vi "Specify Feed Settings Dialog.vi"(11 "error in (no error)":errorcluster) -> (4 "feed name out":string, 6 "feed folderpath out":path, 8 "package destination folderpath out":path, 10 "cancelled?":bool, 15 "error out":errorcluster)   [LabVIEW 2014]
doc: "This VI launches a dialog that prompts the user to add a feed to manage."
uses:
  <vilib>/National Instruments/NIPM API (Beta)/NIPM_API.lvlib
  Specify Feed Settings States.ctl
panel:
  in  "Package Destination Folderpath":path
  in  "Use feed folderpath":bool=TRUE
  in  "Cancel":bool
  in  "OK":bool
  in  "Feed Folderpath":path
  in  "Feed Name":string
  # "Package Destination Folderpath"
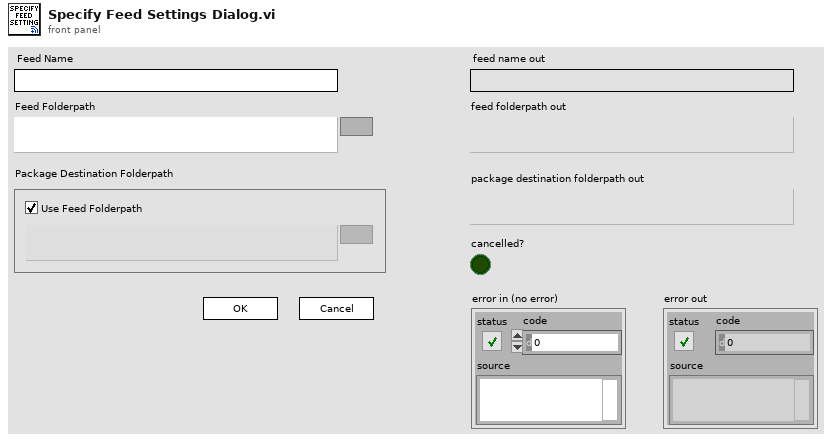
[diagram p1: front panel]
types:
  T1 = typedef "Specify Feed Settings States.ctl" = enum16{"Initialize", "Wait for Event", "Update Display", "Exit"}
  T2 = enum8{"Enabled", "Disabled", "Disabled and Grayed Out"}
  T3 = cluster{"Feed Name":string, "Feed Folderpath":path, "Package Destination Folderpath":path, "Use feed folderpath":bool, "cancelled?":bool}
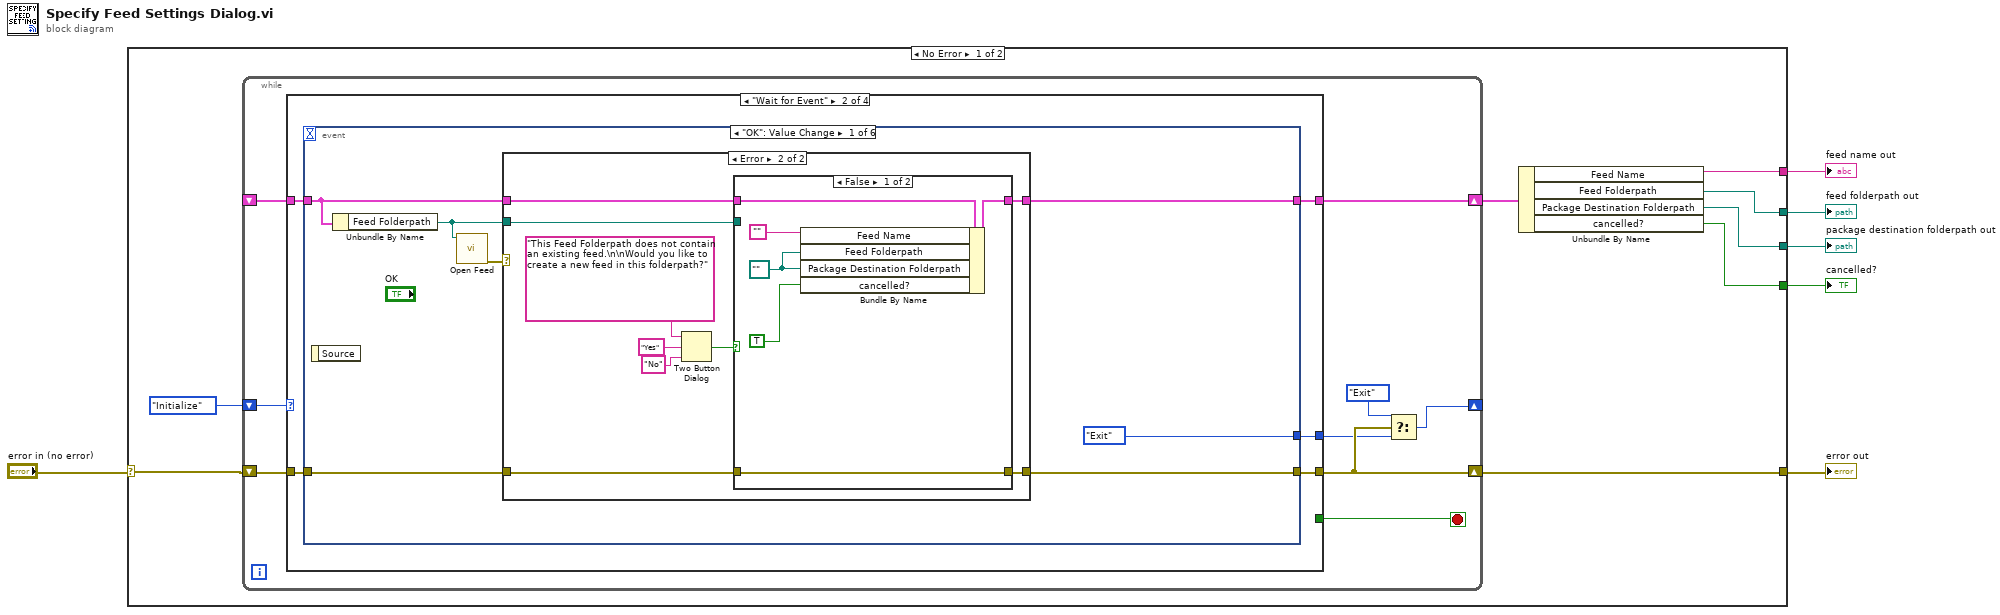
[diagram p0: block diagram]
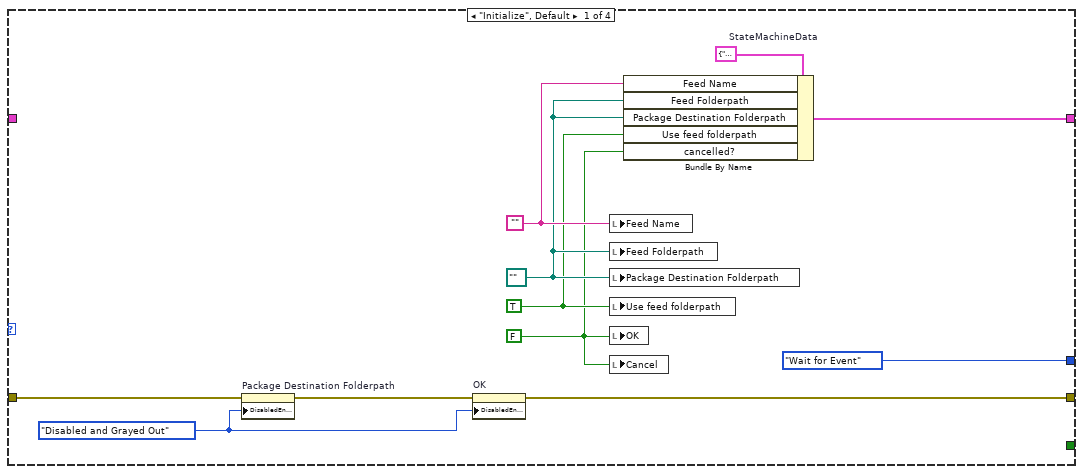
[diagram p2: hidden frame]
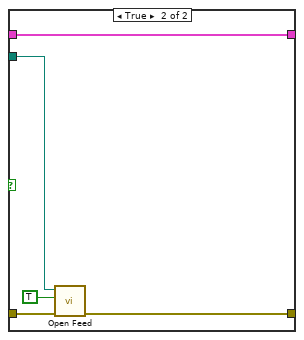
[diagram p4: hidden frame]
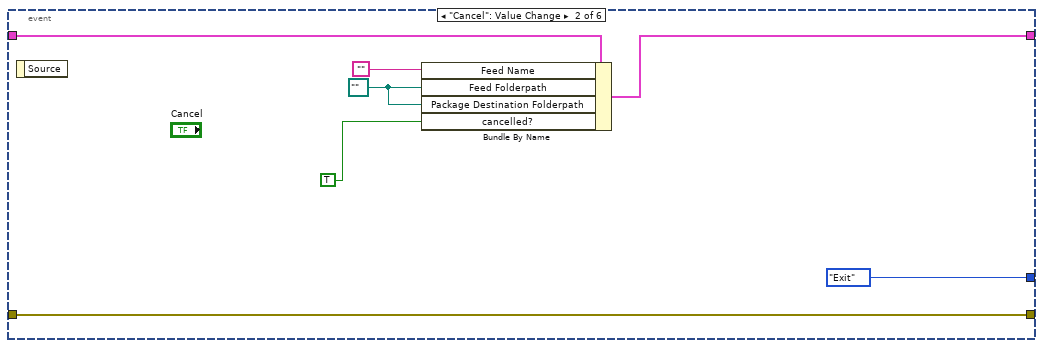
[diagram p5: hidden frame]
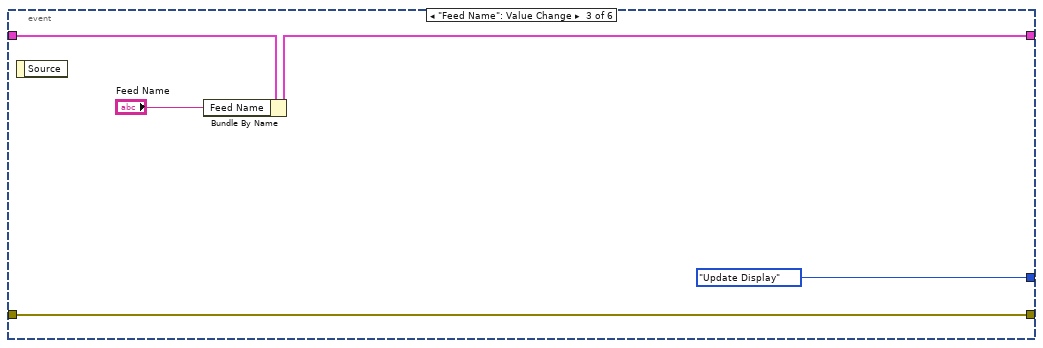
[diagram p6: hidden frame]
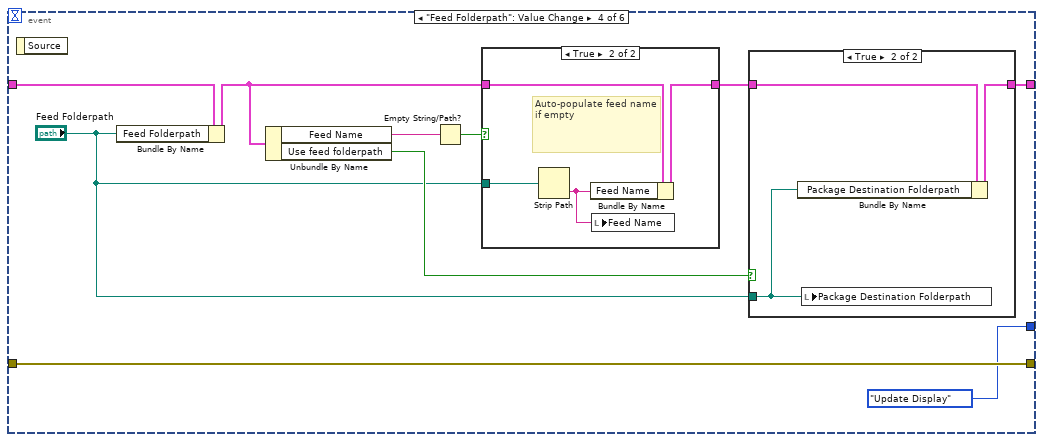
[diagram p7: hidden frame]
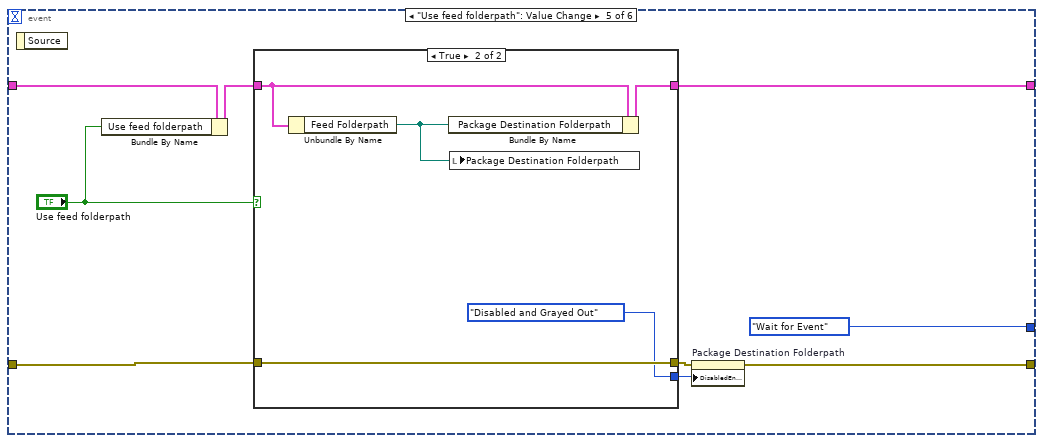
[diagram p10: hidden frame]
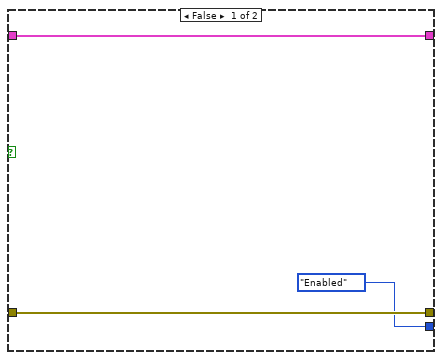
[diagram p11: hidden frame]
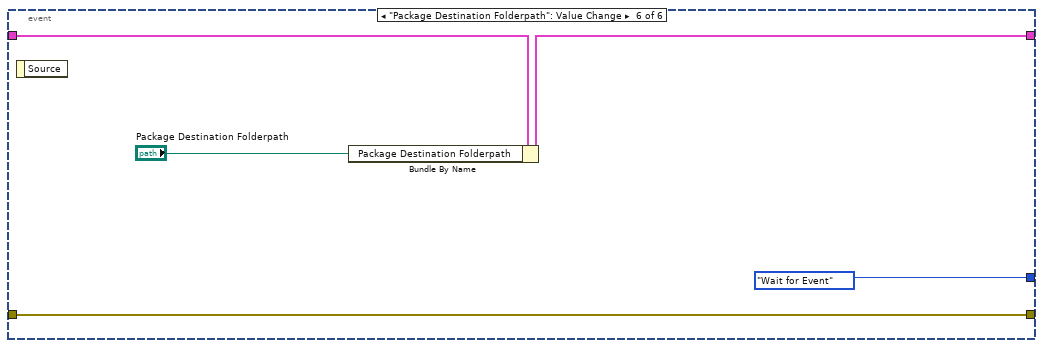
[diagram p12: hidden frame]
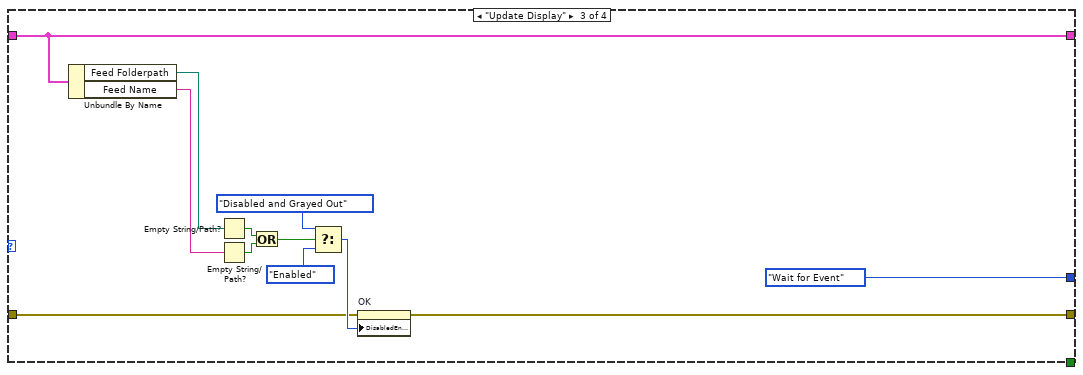
[diagram p13: hidden frame]
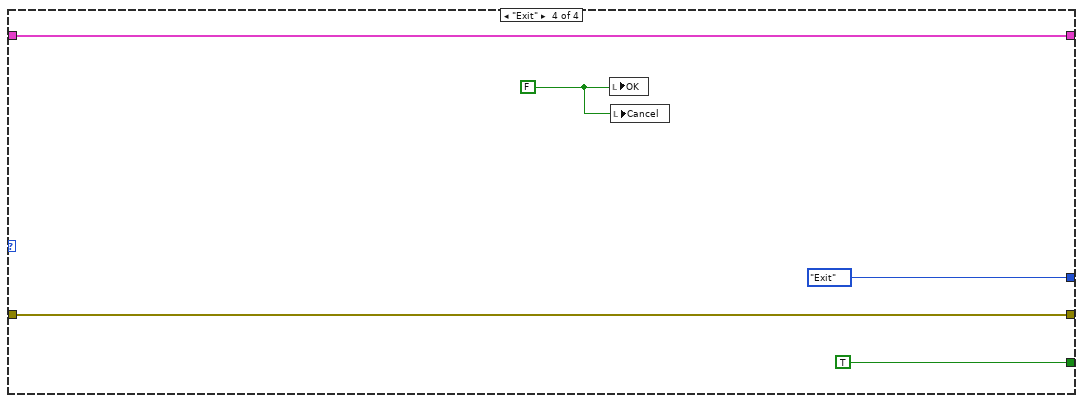
[diagram p14: hidden frame]
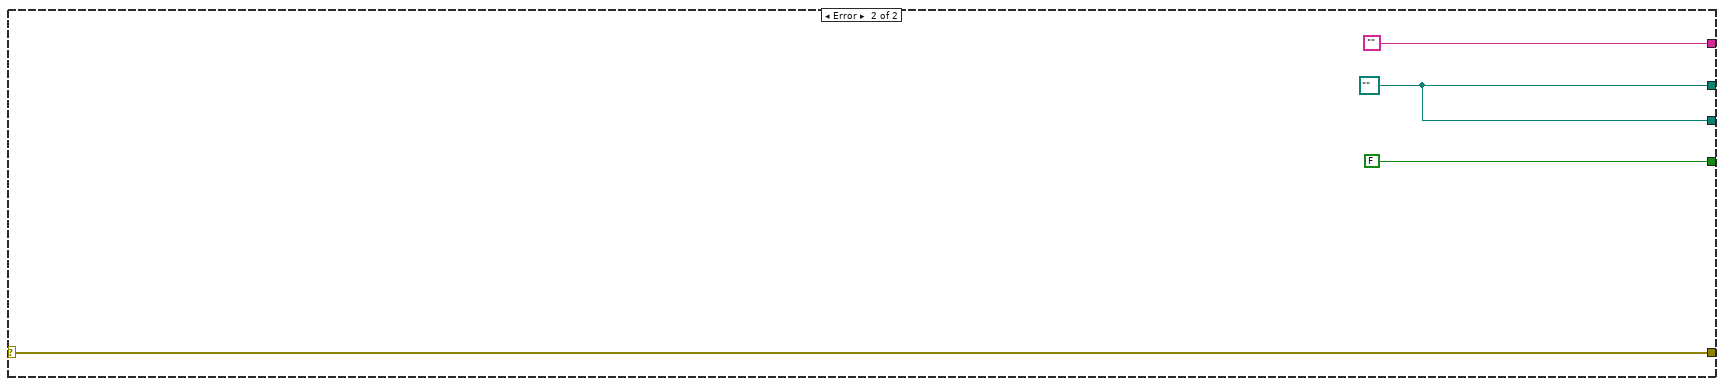
[diagram p15: hidden frame]
diagram:
  n1 = case shown="No Error" "error in (no error)" {
    selector: "error in (no error)" -> [w8 w142]
    tunnel: [w10 FALSE] -> w6
    tunnel: [w12 w139] -> w5
    tunnel: [w11 w139] -> w1
    tunnel: [w14 w142] -> w3
    tunnel: [w7 "" ("Feed Name")] -> w2
    frame No Error {
      n2 = while {
        shift-right: [w18] -> w14
        shift-left: w8 -> [w21]
        shift-right: [w22] -> w13
        shift-left: _ -> [w23]
        shift-right: [w16] -> _
        shift-left: Specify_Feed_Settings_States."Initialize" -> [w20]
        stop <- w19 stop-if-true
        n3 = case shown="\"Wait for Event\"" w20 {
          tunnel: [_ _ _ TRUE] -> w19
          tunnel: w23 -> [_ w39 w125 w136]
          tunnel: [w24 w38 w125 w136] -> w22
          tunnel: w21 -> [w33 w37 w124 w135]
          tunnel: [w30 w36 w123 w135] -> w18
          tunnel: [Specify_Feed_Settings_States."Wait for Event" w35 Specify_Feed_Settings_States."Wait for Event" Specify_Feed_Settings_States."Exit"] -> w15
          frame "Initialize", Default {
            w25 = FALSE ("Use feed folderpath")
            w29 = T3 {"Feed Name"="", "Feed Folderpath"=path "", "Package Destination Folderpath"=path "", "Use feed folderpath"=FALSE, "cancelled?"=FALSE}  # StateMachineData
            w28 = "" ("Feed Name")
            w27 = path "" ("Package Destination Folderpath")
            w26 = TRUE ("Use feed folderpath")
            w31 = T2."Disabled and Grayed Out" ("Disabled")
            n4 = property on="Package Destination Folderpath" class="Path"(error in=w33, "DisabledEnum"=w31) -> (error out=w32:errorcluster)  [unwired: 1 in, 1 out]
            n5 = property on="OK" class="Bool (strict)"(error in=w32, "DisabledEnum"=w31) -> (error out=w30:errorcluster)  [unwired: 1 in, 1 out]
            n6 = local write "Feed Name"(w28) -> ()
            n7 = local write "Feed Folderpath"(w27) -> ()
            n8 = local write "Package Destination Folderpath"(w27) -> ()
            n9 = local write "Use feed folderpath"(w26) -> ()
            n10 = local write "OK"(w25) -> ()
            n11 = local write "Cancel"(w25) -> ()
            n12 = Bundle By Name(cluster=w29, "Feed Name"=w28, "Feed Folderpath"=w27, "Package Destination Folderpath"=w27, "Use feed folderpath"=w26, "cancelled?"=w25) -> (w24:T3)
          }
          frame "Wait for Event" {
            n13 = event shown="[0] \"OK\": Value Change" {
              selector: _ -> [_ _ _ _ _ _]
              dyn-events: _ -> [_ _ _ _ _ _]
              timeout: _ -> [_ _ _ _ _ _]
              tunnel: w39 -> [w45 w75 w80 w90 w108 w121]
              tunnel: [w44 w74 w79 w81 w105 w119] -> w38
              tunnel: w37 -> [w42 w72 w77 w86 w104 w120]
              tunnel: [w41 w72 w77 w86 w107 w120] -> w36
              tunnel: [Specify_Feed_Settings_States."Exit" Specify_Feed_Settings_States."Exit" Specify_Feed_Settings_States."Update Display" Specify_Feed_Settings_States."Update Display" Specify_Feed_Settings_States."Wait for Event" Specify_Feed_Settings_States."Wait for Event"] -> w35
              event "OK": Value Change {
                n14 = event-data() -> ()  [unwired: 1 in, 1 out]
                n15 = Unbundle By Name(w45) -> ("Feed Folderpath"=w43:path)
                n16 = call <vilib>:"Open Feed.vi"("feed folderpath"=w43) -> ("error out"=w46:errorcluster)  [unwired: 8 in, 2 out]
                n17 = case shown="Error" w46 {
                  tunnel: w45 -> [w48 w53]
                  tunnel: [w48 w52] -> w44
                  tunnel: w43 -> [_ w51]
                  tunnel: w42 -> [w47 w50]
                  tunnel: [w47 w49] -> w41
                  frame No Error {
                  }
                  frame Error {
                    n18 = Two Button Dialog(message="This Feed Folderpath does not contain an existing feed.\n\nWould you like to create a new feed in this folderpath?", 1:"No" ("F button name (\"Cancel\")"), 2:"Yes" ("T button name (\"OK\")")) -> (T button?=w54:bool)
                    n19 = case shown="False" w54 {
                      tunnel: w53 -> [w62 w67]
                      tunnel: [w61 w67] -> w52
                      tunnel: w51 -> [_ w66]
                      tunnel: w50 -> [w63 w65]
                      tunnel: [w63 w64] -> w49
                      frame False {
                        w59 = path "" ("Feed Folderpath")
                        n20 = Bundle By Name(cluster=w62, "Feed Name"="", "Feed Folderpath"=w59, "Package Destination Folderpath"=w59, "cancelled?"=TRUE) -> (w61:T3)
                      }
                      frame True {
                        n21 = call <vilib>:"Open Feed.vi"("error in"=w65, "create feed if necessary (F)"=TRUE, "feed folderpath"=w66) -> ("error out"=w64:errorcluster)  [unwired: 6 in, 2 out]
                      }
                    }
                  }
                }
              }
              event "Cancel": Value Change {
                w70 = path "" ("Feed Folderpath")
                n22 = event-data() -> ()  [unwired: 1 in, 1 out]
                n23 = Bundle By Name(cluster=w75, "Feed Name"="", "Feed Folderpath"=w70, "Package Destination Folderpath"=w70, "cancelled?"=TRUE) -> (w74:T3)
              }
              event "Feed Name": Value Change {
                n24 = event-data() -> ()  [unwired: 1 in, 1 out]
                n25 = Bundle By Name(cluster=w80, "Feed Name"="Feed Name") -> (w79:T3)
              }
              event "Feed Folderpath": Value Change {
                n26 = event-data() -> ()  [unwired: 1 in, 1 out]
                n27 = Bundle By Name(cluster=w90, "Feed Folderpath"="Feed Folderpath") -> (w88:T3)
                n28 = Unbundle By Name(w88) -> ("Feed Name"=w89:string, "Use feed folderpath"=w84:bool)
                n29 = Empty String/Path?(string/path=w89) -> (empty?=w87:bool)
                n30 = case shown="True" w87 {
                  tunnel: [w95 w98] -> w82
                  tunnel: w88 -> [w95 w99]
                  tunnel: "Feed Folderpath" -> [_ w97]
                  frame False {
                  }
                  frame True {
                    # "Auto-populate feed name if empty"
                    n31 = Strip Path(path=w97) -> (name=w96:string)  [unwired: 1 out]
                    n32 = Bundle By Name(cluster=w99, "Feed Name"=w96) -> (w98:T3)
                    n33 = local write "Feed Name"(w96) -> ()
                  }
                }
                n34 = case shown="True" w84 {
                  tunnel: "Feed Folderpath" -> [_ w92]
                  tunnel: w82 -> [w91 w94]
                  tunnel: [w91 w93] -> w81
                  frame False {
                  }
                  frame True {
                    n35 = Bundle By Name(cluster=w94, "Package Destination Folderpath"=w92) -> (w93:T3)
                    n36 = local write "Package Destination Folderpath"(w92) -> ()
                  }
                }
              }
              event "Use feed folderpath": Value Change {
                n37 = event-data() -> ()  [unwired: 1 in, 1 out]
                n38 = Bundle By Name(cluster=w108, "Use feed folderpath"="Use feed folderpath") -> (w106:T3)
                n39 = case shown="True" "Use feed folderpath" {
                  tunnel: w106 -> [w109 w116]
                  tunnel: [w109 w115] -> w105
                  tunnel: w104 -> [w111 w114]
                  tunnel: [w111 w114] -> w103
                  tunnel: [T2."Enabled" ("Disabled") T2."Disabled and Grayed Out" ("Disabled")] -> w101
                  frame False {
                  }
                  frame True {
                    n40 = Unbundle By Name(w116) -> ("Feed Folderpath"=w112:path)
                    n41 = Bundle By Name(cluster=w116, "Package Destination Folderpath"=w112) -> (w115:T3)
                    n42 = local write "Package Destination Folderpath"(w112) -> ()
                  }
                }
                n43 = property on="Package Destination Folderpath" class="Path"(error in=w103, "DisabledEnum"=w101) -> (error out=w107:errorcluster)  [unwired: 1 in, 1 out]
              }
              event "Package Destination Folderpath": Value Change {
                n44 = event-data() -> ()  [unwired: 1 in, 1 out]
                n45 = Bundle By Name(cluster=w121, "Package Destination Folderpath"="Package Destination Folderpath") -> (w119:T3)
              }
            }
          }
          frame "Update Display" {
            n46 = Unbundle By Name(w125) -> ("Feed Folderpath"=w132:path, "Feed Name"=w133:string)
            n47 = Empty String/Path?(string/path=w132) -> (empty?=w126:bool)
            n48 = Empty String/Path?(string/path=w133) -> (empty?=w127:bool)
            n49 = Or(x=w126, y=w127) -> (x .or. y?=w128:bool)
            n50 = Select(t=T2."Disabled and Grayed Out" ("Disabled"), s=w128, f=T2."Enabled" ("Disabled")) -> (s? t:f=w129:T2)
            n51 = property on="OK" class="Bool (strict)"(error in=w124, "DisabledEnum"=w129) -> (error out=w123:errorcluster)  [unwired: 1 in, 1 out]
          }
          frame "Exit" {
            w134 = FALSE ("Use feed folderpath")
            n52 = local write "OK"(w134) -> ()
            n53 = local write "Cancel"(w134) -> ()
          }
        }
        n54 = Select(t=Specify_Feed_Settings_States."Exit", s=w18, f=w15) -> (s? t:f=w16:T1)
      }
      n55 = Unbundle By Name(w13) -> ("Feed Name"=w7:string, "Feed Folderpath"=w12:path, "Package Destination Folderpath"=w11:path, "cancelled?"=w10:bool)
    }
    frame Error {
      w139 = path "" ("Feed Folderpath")
    }
  }
  "cancelled?" <- w6
  "feed folderpath out" <- w5
  "feed name out" <- w2
  "error out" <- w3
  "package destination folderpath out" <- w1
